vi "Read Path.vi"(8 "error in (no error)":errorcluster, 11 "Logging Txt in":refnum<class "Logging Txt.lvclass">) -> (0 "error out":errorcluster, 2 "Path":path, 3 "Logging Txt out":refnum<class "Logging Txt.lvclass">)   [LabVIEW 2020, in "Logging Txt.lvlib" / "Logging Txt.lvclass"]
uses:
  Logging Txt.lvclass
  Logging Txt.lvclass/Logging Txt.ctl
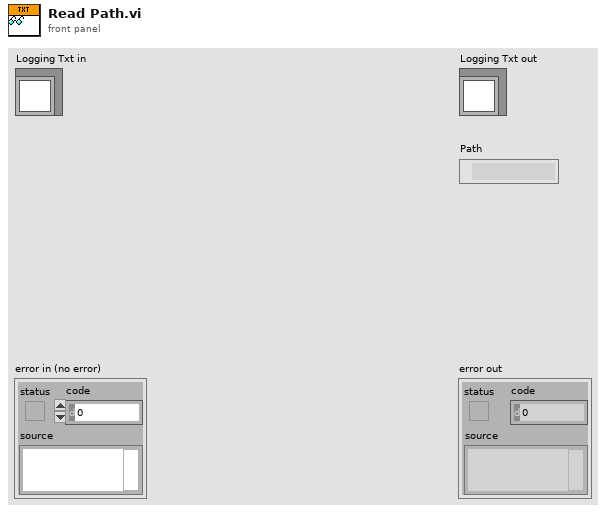
[diagram p1: front panel]
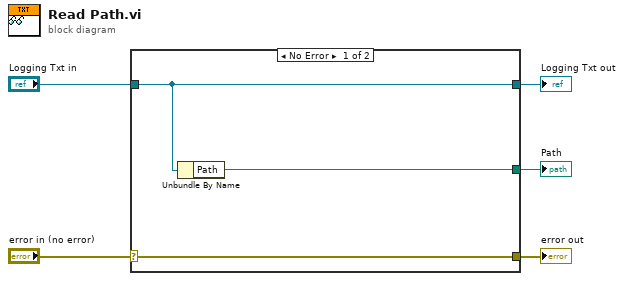
[diagram p0: block diagram]
diagram:
  n1 = case shown="No Error" "error in (no error)" {
    selector: "error in (no error)" -> [w8 w9]
    tunnel: [w8 w9] -> w4
    tunnel: [w7 w10] -> w2
    tunnel: "Logging Txt in" -> [w7 w10]
    tunnel: [w6 _] -> w1
    frame No Error {
      n2 = Unbundle By Name(w7) -> ("Path"=w6:path)
    }
    frame Error {
    }
  }
  "error out" <- w4
  "Logging Txt out" <- w2
  "Path" <- w1
